vi "Warnings.vi"() -> ()   [LabVIEW 2014]
panel:
  out "Warning Text":string
  out "Warning?":bool
  in  "Min Temp":dbl
  in  "Max Temp":dbl
  in  "Current Temp":dbl
  # "You must create a portion of a larger project. The lead developer gives you the inputs of the VI, the\nalgorithm, and the expected outputs. Create and document a VI based on the given design."
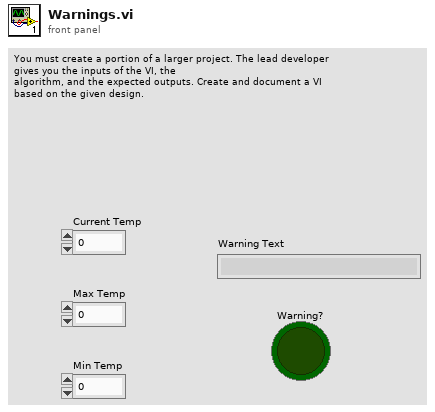
[diagram p1: front panel]
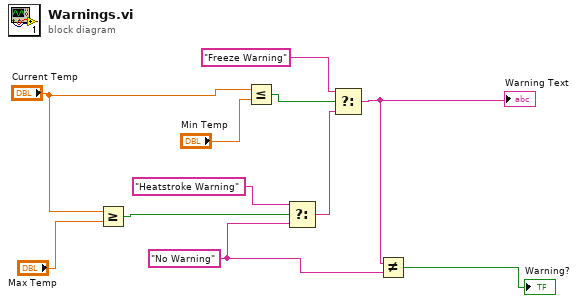
[diagram p0: block diagram]
diagram:
  w1 = "No Warning"
  n1 = Greater Or Equal?(x="Current Temp", y="Max Temp") -> (x >= y?=w10:bool)
  n2 = Less Or Equal?(x="Current Temp", y="Min Temp") -> (x <= y?=w4:bool)
  n3 = Select(t="Heatstroke Warning", s=w10, f=w1) -> (s? t:f=w5:string)
  n4 = Select(t="Freeze Warning", s=w4, f=w5) -> (s? t:f=w2:string)
  "Warning Text" <- w2
  n5 = Not Equal?(x=w2, y=w1) -> (x != y?=→"Warning?":bool)
